vi "Get Temperature.vi"(6 "Channel":i32, 8 "error in (no error)":errorcluster, 11 "Instrument.MNK_TC in":refnum<class "Instrument.MNK_TC.lvclass">) -> (0 "error out":errorcluster, 1 "Status":variant, 2 "Temperature (K)":dbl, 3 "Instrument.MNK_TC out":refnum<class "Instrument.MNK_TC.lvclass">, 4 "Finished?":bool)   [LabVIEW 2016, in "Instrument.MNK_TC.lvclass"]
uses:
  Instrument.MNK_TC.lvclass
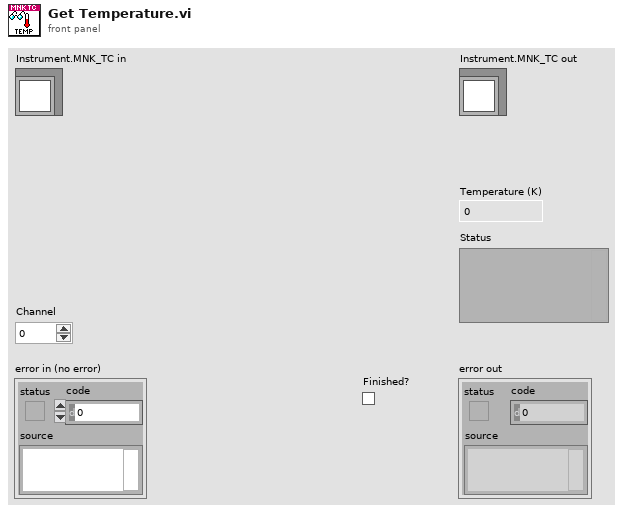
[diagram p1: front panel]
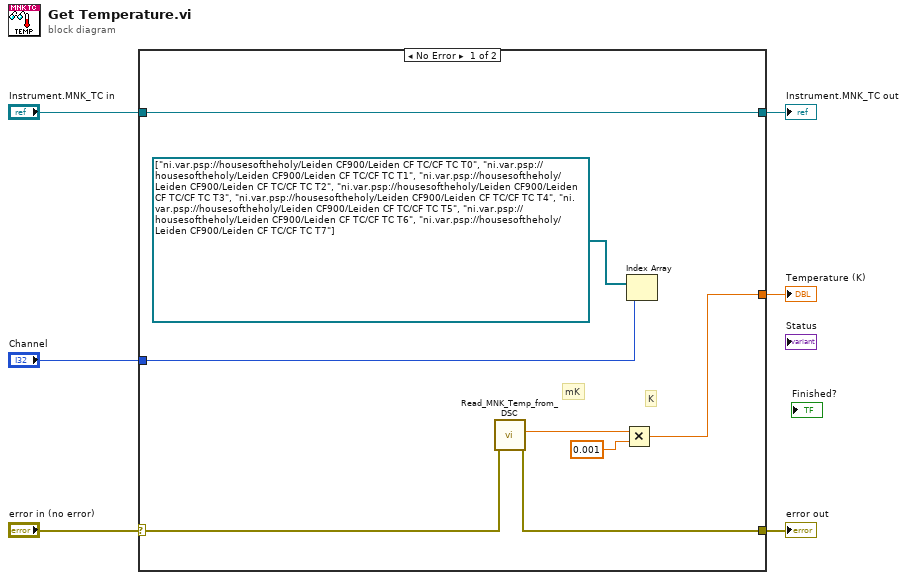
[diagram p0: block diagram]
diagram:
  n1 = case shown="No Error" "error in (no error)" {
    selector: "error in (no error)" -> [w12 w15]
    tunnel: [w11 w15] -> w5
    tunnel: [w14 w16] -> w4
    tunnel: "Instrument.MNK_TC in" -> [w14 w16]
    tunnel: [w8 _] -> w2
    tunnel: "Channel" -> [w7 _]
    frame No Error {
      # "K"
      # "mK"
      n2 = call "Read_MNK_Temp_from_DSC.vi"("Error in (no error)"=w12) -> ("Error out"=w11:errorcluster, "Temp"=w13:dbl)  [unwired: 9 in]
      n3 = Multiply(x=w13, y=0.001) -> (x*y=w8:dbl)
      n4 = Index Array(array=refnum<k21>[] ["ni.var.psp://housesoftheholy/Leiden CF900/Leiden CF TC/CF TC T0", "ni.var.psp://housesoftheholy/Leiden CF900/Leiden CF TC/CF TC T1", "ni.var.psp://housesoftheholy/Leiden CF900/Leiden CF TC/CF TC T2", "ni.var.psp://housesoftheholy/Leiden CF900/Leiden CF TC/CF TC T3", "ni.var.psp://housesoftheholy/Leiden CF900/Leiden CF TC/CF TC T4", "ni.var.psp://housesoftheholy/Leiden CF900/Leiden CF TC/CF TC T5", "ni.var.psp://housesoftheholy/Leiden CF900/Leiden CF TC/CF TC T6", "ni.var.psp://housesoftheholy/Leiden CF900/Leiden CF TC/CF TC T7"] ("dbl var"), index=w7) -> ()  [unwired: 1 out]
    }
    frame Error {
    }
  }
  "error out" <- w5
  "Instrument.MNK_TC out" <- w4
  "Temperature (K)" <- w2
